vi "Populate Subpanels.vi"(8 "error in (no error)":errorcluster, 9 "View Labels (optional)":string[](array[string]), 10 "Views":refnum<class "Message Enqueuer.lvclass">[](array[class]), 11 "TabbedViewManager In":refnum<class "TabbedViewManager.lvclass">) -> (0 "error out":errorcluster, 3 "TabbedViewManager Out":refnum<class "TabbedViewManager.lvclass">)   [LabVIEW 2015, in "TabbedViewManager.lvlib" / "TabbedViewManager.lvclass"]
doc: "<License>\nCopyright © 2017 Composed Systems, LLC | All rights reserved\nwww.composed.io\n\nAuthor: Ethan Stern <ethan.stern@composed.io>\n\nThis software is provided \"AS IS\" WITHOUT WARRANTIES, either express or implied, AND IS FOR EDUCATIONAL PURPOSES ONLY.\n</License>"
uses:
  TabbedViewManager.lvclass
  <vilib>/ActorFramework/Message Enqueuer/Message Enqueuer.lvclass
  TabbedViewManager.lvclass/TabbedViewManager.ctl
  Framework/IViewable/IViewable Messages/Insert Front Panel Msg/Insert Front Panel Msg.lvclass/Insert Front Panel Msg.ctl
  <vilib>/ActorFramework/Message Enqueuer/Message Enqueuer.lvclass/Message Enqueuer.ctl
  <vilib>/ActorFramework/Message Enqueuer/Enqueue.vi
  <vilib>/ActorFramework/Message Priority Queue/Priority Enqueue.vi
  Framework/IViewManager/IViewManager/IViewManager.lvclass
  Framework/IViewable/IViewable Messages/Insert Front Panel Msg/Insert Front Panel Msg.lvclass
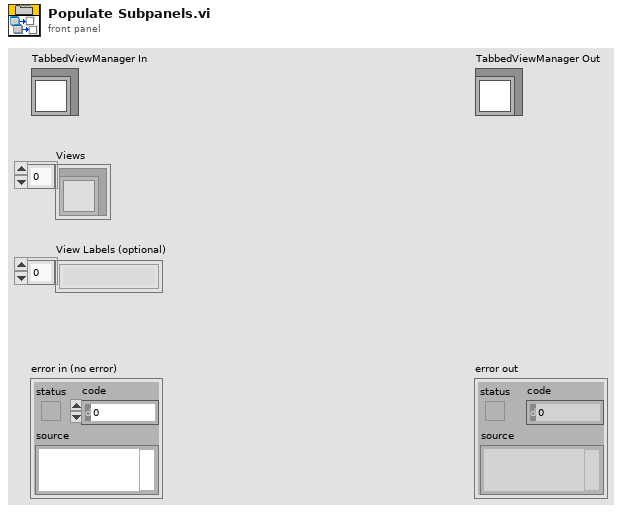
[diagram p1: front panel]
types:
  T1 = enum32{"1", "2", "3", "4", "5", "6", "7", "8", "9", "10"}
  T2 = typedef "IViewable.lvlib/ProtectedSubpanel.lvclass/Protected Subpanel Reference.ctl" = refnum<data-value>
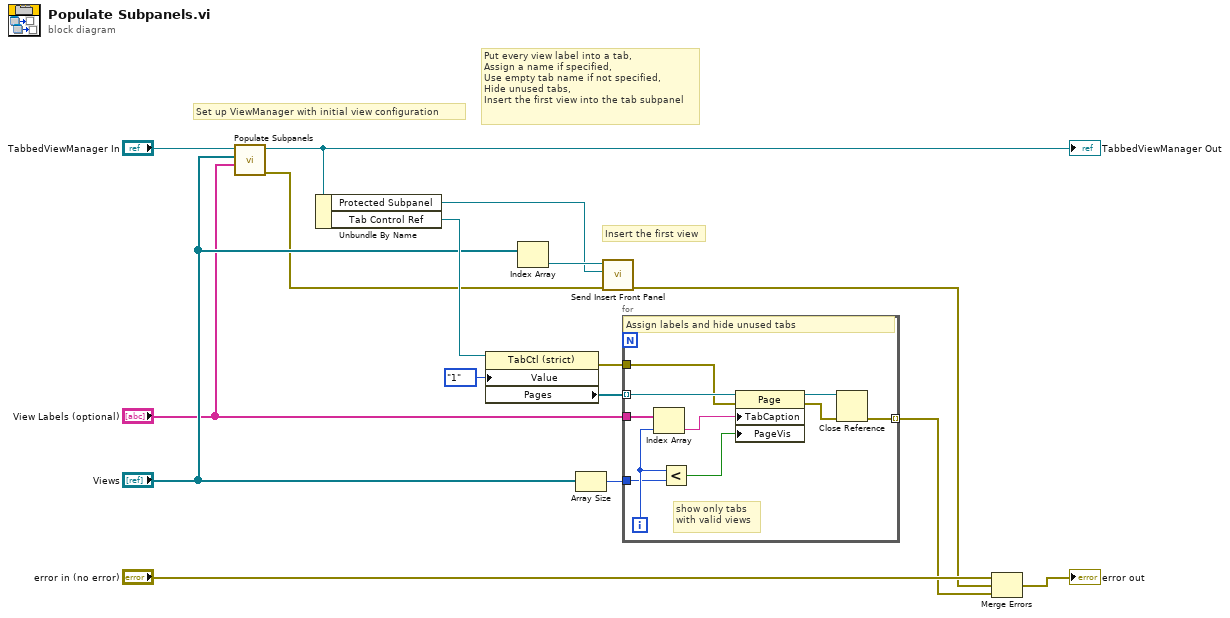
[diagram p0: block diagram]
diagram:
  # "Set up ViewManager with initial view configuration"
  # "Put every view label into a tab,\nAssign a name if specified,\nUse empty tab name if not specified,\nHide unused tabs,\nInsert the first view into the tab subpanel"
  # "Insert the first view"
  n1 = call-parent "Populate Subpanels.vi"("View Labels (optional)"="View Labels (optional)", "Views"="Views", "IViewManager In"="TabbedViewManager In") -> ("error out"=w2:errorcluster, "IViewManager Out"=w5:refnum<class "TabbedViewManager.lvclass">)  [unwired: 7 in]
  "TabbedViewManager Out" <- w5
  n2 = Unbundle By Name(w5) -> ("Protected Subpanel"=w10:T2, "Tab Control Ref"=w11:refnum<vi>)
  n3 = property class="TabCtl (strict)"(reference=w11, "Value"=T1."1") -> (error out=w13:errorcluster, "Pages"=w15:refnum<vi>[])  [unwired: 1 in, 1 out]
  n4 = Index Array(array="Views") -> (element=w12:refnum<class "Message Enqueuer.lvclass">)  [unwired: 1 in]
  n5 = Array Size(array="Views") -> (size(s)=w14:i32)
  n6 = call "Send Insert Front Panel.vi"("error in (no error)"=w2, "Protected Subpanel"=w10, "Message Enqueuer"=w12) -> ("error out"=w3:errorcluster)  [unwired: 7 in, 1 out]
  n7 = for {
    tunnel: w15 -> [w26] mode=indexing
    tunnel: "View Labels (optional)" -> [w25]
    tunnel: w14 -> [w22]
    tunnel: w13 -> [w18]
    tunnel: [w17] -> w4 mode=indexing
    i -> [w23]
    # "show only tabs\nwith valid views"
    # "Assign labels and hide unused tabs"
    n8 = Index Array(array=w25, index=w23) -> (element=w24:string)
    n9 = Less?(x=w23, y=w22) -> (x < y?=w21:bool)
    n10 = property class="Page"(reference=w26, error in=w18, "TabCaption"=w24, "PageVis"=w21) -> (reference out=w20:refnum<vi>, error out=w19:errorcluster)
    n11 = Close Reference(reference=w20, error in (no error)=w19) -> (error out=w17:errorcluster)
  }
  n12 = Merge Errors("error in (no error)", w3, w4) -> (→"error out":errorcluster)
